vi "AT_Leds_UI.vi"(1 "Array_Test":T1(array[cluster])=[{"Accion"="Leer", "Time ms"=100, "Valor Esperado"="00 00 00 00 00 00", "ERD Number"=61467, "Data_To_Write"=""}, {"Accion"="Escribir", "Time ms"=100, "Valor Esperado"="", "ERD Number"=61467, "Data_To_Write"="01 00 00 00 00 00"}, {"Accion"="N/A", "Time ms"=1000, "Valor Esperado"="", "ERD Number"=0, "Data_To_Write"=""}, {"Accion"="Escribir", "Time ms"=100, "Valor Esperado"="", "ERD Number"=61467, "Data_To_Write"="02 00 00 00 00 00"}, {"Accion"="N/A", "Time ms"=1000, "Valor Esperado"="", "ERD Number"=0, "Data_To_Write"=""}, {"Accion"="Escribir", "Time ms"=100, "Valor Esperado"="", "ERD Number"=61467, "Data_To_Write"="03 00 00 00 00 00"}, {"Accion"="N/A", "Time ms"=1000, "Valor Esperado"="", "ERD Number"=0, "Data_To_Write"=""}, {"Accion"="Escribir", "Time ms"=100, "Valor Esperado"="", "ERD Number"=61467, "Data_To_Write"="04 00 00 00 00 00"}, {"Accion"="N/A", "Time ms"=1000, "Valor Esperado"="", "ERD Number"=0, "Data_To_Write"=""}, {"Accion"="Escribir", "Time ms"=100, "Valor Esperado"="", "ERD Number"=61467, "Data_To_Write"="05 00 00 00 00 00"}, {"Accion"="N/A", "Time ms"=1000, "Valor Esperado"="", "ERD Number"=0, "Data_To_Write"=""}, {"Accion"="Escribir", "Time ms"=100, "Valor Esperado"="", "ERD Number"=61467, "Data_To_Write"="07 00 00 00 00 00"}, {"Accion"="N/A", "Time ms"=1000, "Valor Esperado"="", "ERD Number"=0, "Data_To_Write"=""}, {"Accion"="Escribir", "Time ms"=100, "Valor Esperado"="", "ERD Number"=61467, "Data_To_Write"="08 00 00 00 00 00"}, {"Accion"="N/A", "Time ms"=1000, "Valor Esperado"="", "ERD Number"=0, "Data_To_Write"=""}, {"Accion"="Escribir", "Time ms"=100, "Valor Esperado"="", "ERD Number"=61467, "Data_To_Write"="09 00 00 00 00 00"}, {"Accion"="N/A", "Time ms"=1000, "Valor Esperado"="", "ERD Number"=0, "Data_To_Write"=""}, {"Accion"="Escribir", "Time ms"=100, "Valor Esperado"="", "ERD Number"=61467, "Data_To_Write"="0A 00 00 00 00 00"}, {"Accion"="N/A", "Time ms"=1000, "Valor Esperado"="", "ERD Number"=0, "Data_To_Write"=""}, {"Accion"="Escribir", "Time ms"=100, "Valor Esperado"="", "ERD Number"=61467, "Data_To_Write"="0B 00 00 00 00 00"}, {"Accion"="N/A", "Time ms"=1000, "Valor Esperado"="", "ERD Number"=0, "Data_To_Write"=""}, {"Accion"="Escribir", "Time ms"=100, "Valor Esperado"="", "ERD Number"=61467, "Data_To_Write"="0C 00 00 00 00 00"}, {"Accion"="N/A", "Time ms"=1000, "Valor Esperado"="", "ERD Number"=0, "Data_To_Write"=""}, {"Accion"="Escribir", "Time ms"=100, "Valor Esperado"="", "ERD Number"=61467, "Data_To_Write"="0E 00 00 00 00 00"}, {"Accion"="N/A", "Time ms"=1000, "Valor Esperado"="", "ERD Number"=0, "Data_To_Write"=""}, {"Accion"="Escribir", "Time ms"=100, "Valor Esperado"="", "ERD Number"=61467, "Data_To_Write"="0F 00 00 00 00 00"}, {"Accion"="N/A", "Time ms"=1000, "Valor Esperado"="", "ERD Number"=0, "Data_To_Write"=""}, {"Accion"="Escribir", "Time ms"=100, "Valor Esperado"="", "ERD Number"=61467, "Data_To_Write"="00 00 00 00 00 00"}] {"ERD Number" format="%.0x"; "Time ms" min=100}) -> (0 "Array_Test 2":T1(array[cluster])=[{"Accion"="Leer", "Time ms"=100, "Valor Esperado"="00 00 00 00 00 00", "ERD Number"=61467, "Data_To_Write"=""}, {"Accion"="Escribir", "Time ms"=100, "Valor Esperado"="", "ERD Number"=61467, "Data_To_Write"="01 00 00 00 00 00"}, {"Accion"="N/A", "Time ms"=1000, "Valor Esperado"="", "ERD Number"=0, "Data_To_Write"=""}, {"Accion"="Escribir", "Time ms"=100, "Valor Esperado"="", "ERD Number"=61467, "Data_To_Write"="02 00 00 00 00 00"}, {"Accion"="N/A", "Time ms"=1000, "Valor Esperado"="", "ERD Number"=0, "Data_To_Write"=""}, {"Accion"="Escribir", "Time ms"=100, "Valor Esperado"="", "ERD Number"=61467, "Data_To_Write"="03 00 00 00 00 00"}, {"Accion"="N/A", "Time ms"=1000, "Valor Esperado"="", "ERD Number"=0, "Data_To_Write"=""}, {"Accion"="Escribir", "Time ms"=100, "Valor Esperado"="", "ERD Number"=61467, "Data_To_Write"="04 00 00 00 00 00"}, {"Accion"="N/A", "Time ms"=1000, "Valor Esperado"="", "ERD Number"=0, "Data_To_Write"=""}, {"Accion"="Escribir", "Time ms"=100, "Valor Esperado"="", "ERD Number"=61467, "Data_To_Write"="05 00 00 00 00 00"}, {"Accion"="N/A", "Time ms"=1000, "Valor Esperado"="", "ERD Number"=0, "Data_To_Write"=""}, {"Accion"="Escribir", "Time ms"=100, "Valor Esperado"="", "ERD Number"=61467, "Data_To_Write"="07 00 00 00 00 00"}, {"Accion"="N/A", "Time ms"=1000, "Valor Esperado"="", "ERD Number"=0, "Data_To_Write"=""}, {"Accion"="Escribir", "Time ms"=100, "Valor Esperado"="", "ERD Number"=61467, "Data_To_Write"="08 00 00 00 00 00"}, {"Accion"="N/A", "Time ms"=1000, "Valor Esperado"="", "ERD Number"=0, "Data_To_Write"=""}, {"Accion"="Escribir", "Time ms"=100, "Valor Esperado"="", "ERD Number"=61467, "Data_To_Write"="09 00 00 00 00 00"}, {"Accion"="N/A", "Time ms"=1000, "Valor Esperado"="", "ERD Number"=0, "Data_To_Write"=""}, {"Accion"="Escribir", "Time ms"=100, "Valor Esperado"="", "ERD Number"=61467, "Data_To_Write"="0A 00 00 00 00 00"}, {"Accion"="N/A", "Time ms"=1000, "Valor Esperado"="", "ERD Number"=0, "Data_To_Write"=""}, {"Accion"="Escribir", "Time ms"=100, "Valor Esperado"="", "ERD Number"=61467, "Data_To_Write"="0B 00 00 00 00 00"}, {"Accion"="N/A", "Time ms"=1000, "Valor Esperado"="", "ERD Number"=0, "Data_To_Write"=""}, {"Accion"="Escribir", "Time ms"=100, "Valor Esperado"="", "ERD Number"=61467, "Data_To_Write"="0C 00 00 00 00 00"}, {"Accion"="N/A", "Time ms"=1000, "Valor Esperado"="", "ERD Number"=0, "Data_To_Write"=""}, {"Accion"="Escribir", "Time ms"=100, "Valor Esperado"="", "ERD Number"=61467, "Data_To_Write"="0E 00 00 00 00 00"}, {"Accion"="N/A", "Time ms"=1000, "Valor Esperado"="", "ERD Number"=0, "Data_To_Write"=""}, {"Accion"="Escribir", "Time ms"=100, "Valor Esperado"="", "ERD Number"=61467, "Data_To_Write"="0F 00 00 00 00 00"}, {"Accion"="N/A", "Time ms"=1000, "Valor Esperado"="", "ERD Number"=0, "Data_To_Write"=""}, {"Accion"="Escribir", "Time ms"=100, "Valor Esperado"="", "ERD Number"=61467, "Data_To_Write"="00 00 00 00 00 00"}] {"ERD Number" format="%.0x"; "Time ms" min=100})   [LabVIEW 2021]
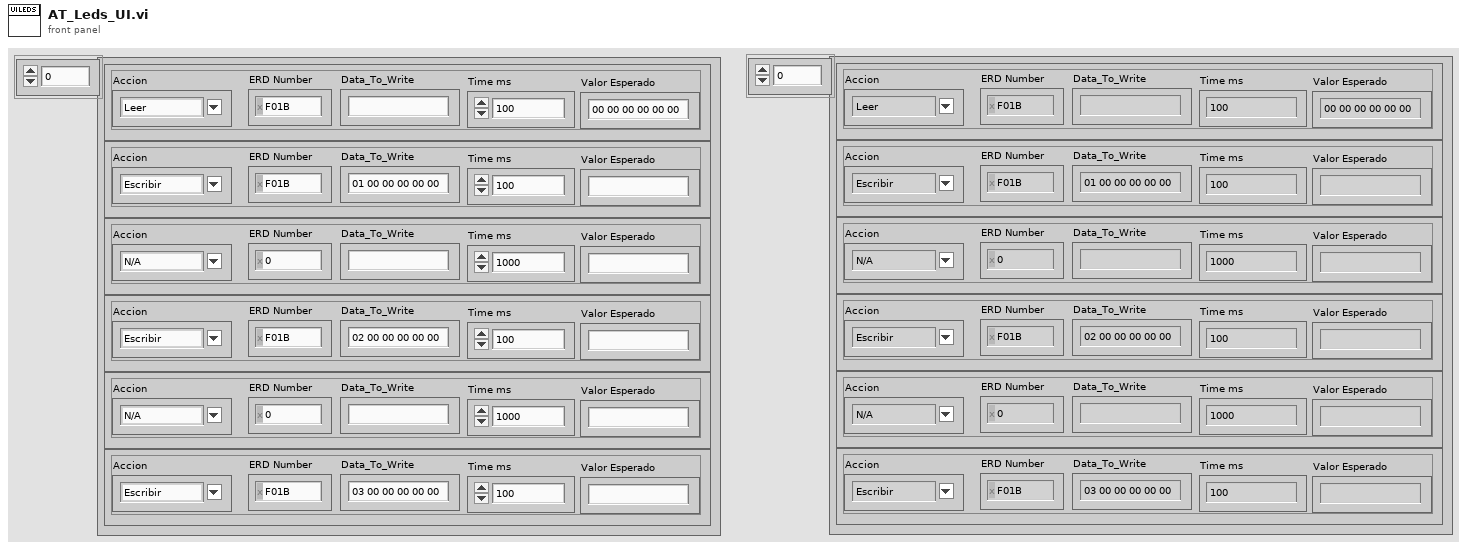
[diagram p1: front panel]
types:
  T1 = cluster{"Accion":string, "Time ms":u32, "Valor Esperado":string, "ERD Number":u16, "Data_To_Write":string}[]
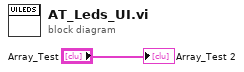
[diagram p0: block diagram]
diagram:
  "Array_Test 2" <- "Array_Test"
